vi "Stepper Write.vi"(6 "Set Acceleration (0 to disable)":i16, 7 "Stepper #":u8, 8 "Error In":errorcluster, 9 "Set Speed (Steps per Second)":i16=100, 10 "# of Steps to Move":i16, 11 "ChipKit Resource":T1={"COM Port"="", "Board Type"=enum."ChipKit uC32", "Connection Type"=enum."USB / Serial", "Baud Rate (115200)"=15, "Bytes Per Packet (15)"=15, "DI Port Num Pins"=0, "DO Port Num Pins"=0}) -> (0 "Error Out":errorcluster, 3 "ChipKit Resource":T1={"COM Port"="", "Board Type"=enum."ChipKit uC32", "Connection Type"=enum."USB / Serial", "Baud Rate (115200)"=15, "Bytes Per Packet (15)"=15, "DI Port Num Pins"=0, "DO Port Num Pins"=0})   [LabVIEW 2011, in "LabVIEW Interface for ChipKit.lvlib"]
doc: "Specify the speed and number of steps to move the stepper motor. Optionally, specify acceleration in steps per second per second."
uses:
  LabVIEW Interface for ChipKit.lvlib
  Private/Type Defs/Chipkit Resource.ctl
  Private/Type Defs/Board Type.ctl
  Private/Type Defs/Connection Type.ctl
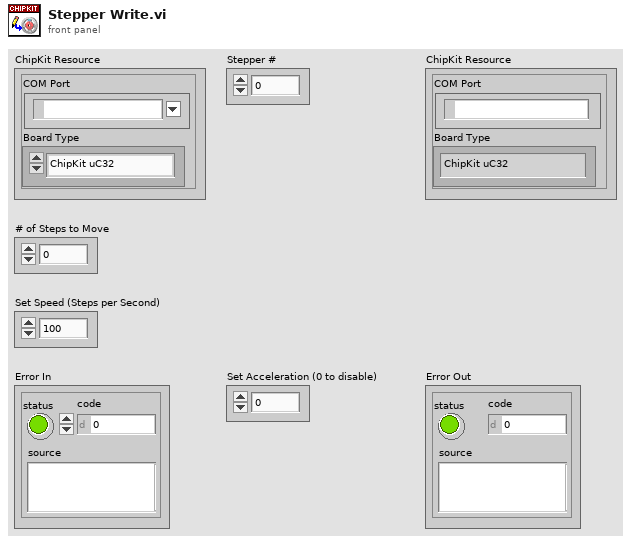
[diagram p1: front panel]
types:
  T1 = typedef "LabVIEW Interface for ChipKit.lvlib/Chipkit Resource.ctl" = cluster{"COM Port":refnum<visa-resource-name>, "Board Type":T2, "Connection Type":T3, "Baud Rate (115200)":u32, "Bytes Per Packet (15)":u32, "DI Port Num Pins":i32, "DO Port Num Pins":i32}
  T2 = typedef "LabVIEW Interface for ChipKit.lvlib/Board Type.ctl" = enum16{"ChipKit uC32", "ChipKit Uno32", "ChipKit Max32"}
  T3 = typedef "LabVIEW Interface for ChipKit.lvlib/Connection Type.ctl" = enum8{"USB / Serial", "XBEE", "BlueSmirf (Bluetooth)"}
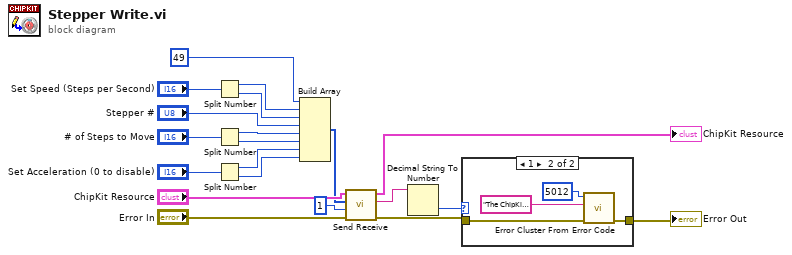
[diagram p0: block diagram]
diagram:
  n1 = Split Number(x="Set Speed (Steps per Second)") -> (hi(x)=w17:u8, lo(x)=w16:u8)
  n2 = Split Number(x="# of Steps to Move") -> (hi(x)=w14:u8, lo(x)=w13:u8)
  n3 = Split Number(x="Set Acceleration (0 to disable)") -> (hi(x)=w11:u8, lo(x)=w10:u8)
  n4 = Build Array(u8 49, w17, w16, "Stepper #", w14, w13, w11, w10) -> (w6:u8[])
  n5 = call "Send Receive.vi"("Error In"="Error In", "Bytes To Read (0)"=u8 1, "Data"=w6, "ChipKit Resource"="ChipKit Resource") -> ("Error Out"=w3:errorcluster, "Read Buffer"=w5:string, "ChipKit Resource"=→"ChipKit Resource":T1)  [unwired: 5 in]
  n6 = Decimal String To Number(string=w5) -> (number=w9:i32)  [unwired: 2 in, 1 out]
  n7 = case shown="1" w9 {
    tunnel: w3 -> [w21 w23]
    tunnel: [w21 w22] -> w8
    frame 0, Default {
    }
    frame 1 {
      n8 = call <vilib>:"Error Cluster From Error Code.vi"("error in (no error)"=w23, "error message (\"\")"="The ChipKit firmware returned an error when attempting to write the stepper motor value." ("source"), "error code (0)"=5012) -> ("error out"=w22:errorcluster)  [unwired: 6 in]
    }
  }
  "Error Out" <- w8
